vi "Client Output Test.vi"() -> (0 "Error Out":errorcluster, 2 "Pass?":bool)   [LabVIEW 2013, in "OPC UA Client Tests.lvlib"]
doc: "Test functionality of output.vi of the OPC UA Client runtime.lvclass"
uses:
  OPC UA Client Tests.lvlib
  <vilib>/NI/Tag Bus Module Framework/channel/channel classification.ctl
  module/execution/OPC UA Client runtime.lvclass/OPC UA Client runtime.ctl
  module/execution/OPC UA Client runtime.lvclass
  <vilib>/NI/Tag Bus Module Framework/channel/TBM channel.lvclass
panel:
  out "Individual Tests":bool[](array[boolean])
  # "13"
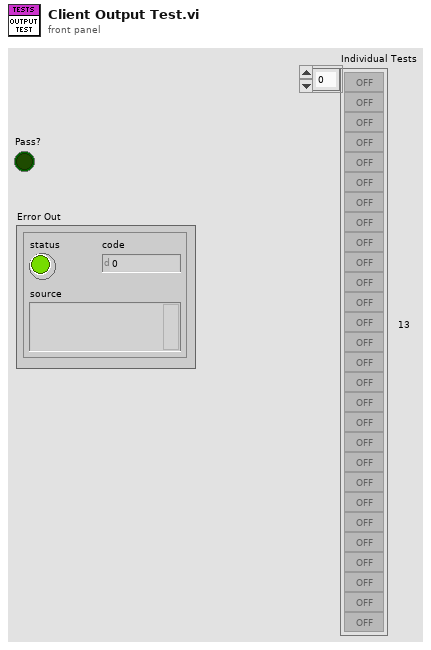
[diagram p1: front panel]
types:
  T1 = typedef "TBM channel.lvclass/channel classification.ctl" = enum16{"input data", "output data", "processing parameter", "processing result"}
  T2 = typedef "TBM channel.lvclass/data tables.ctl" = cluster{"input data":T3, "processing parameter":T3, "processing result":T3, "output data":T3}
  T3 = typedef "tag bus.lvlib/dictionary table pair.ctl" = cluster{"data dictionary":refnum<class "data dictionary.lvclass">, "data table":T4}
  T4 = typedef "tag bus.lvlib/data table.lvlib/data table.ctl" = cluster{"Double":dbl[], "Single":sgl[], "I64":i64[], "I32":i32[], "I16":i16[], "I8":i8[], "U64":u64[], "U32":u32[], "U16":u16[], "U8":u8[], "Boolean":bool[], "String":string[], "Array of Double":cluster{"DBL Array":dbl[]}[], "Array of Single":cluster{"SGL Array":sgl[]}[], "Array of I64":cluster{"I64 Array":i64[]}[], "Array of I32":cluster{"I32 Array":i32[]}[], "Array of I16":cluster{"I16 Array":i16[]}[], "Array of I8":cluster{"I8 Array":i8[]}[], "Array of U64":cluster{"U64 Array":u64[]}[], "Array of U32":cluster{"U32 Array":u32[]}[], "Array of U16":cluster{"U16 Array":u16[]}[], "Array of U8":cluster{"U8 Array":u8[]}[], "Array of Boolean":cluster{"Boolean Array":bool[]}[], "Array of String":cluster{"String Array":string[]}[]}
  T5 = typedef "OPC UA Client configuration.lvclass/Line.ctl" = cluster{"channel":refnum<class "TBM channel.lvclass">, "Node Path":string, "OPC UA Data Type":T6}
  T6 = typedef "OPC UA Client configuration.lvclass/OPC UA Data Type.ctl" = u16
  T7 = typedef "tag bus.lvlib/tag descriptor.lvclass/Data Type.ctl" = enum16{"Double", "Single", "I64", "I32", "I16", "I8", "U64", "U32", "U16", "U8", "Boolean", "String", "Array of Double", "Array of Single", "Array of I64", "Array of I32", "Array of I16", "Array of I8", "Array of U64", "Array of U32", "Array of U16", "Array of U8", "Array of Boolean", "Array of String"}
  T8 = cluster{"DCAF Data Type":T7, "Index":i32, "Node Path":string, "OPC UA Data Type":T6}[]
  T9 = cluster{"Node Path":string, "Flattened Data":string}[]
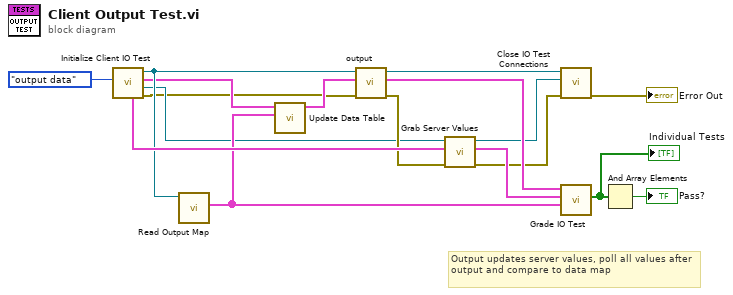
[diagram p0: block diagram]
diagram:
  # "Output updates server values, poll all values after output and compare to data map"
  n1 = call "Initialize Client IO Test.vi"("channel classification"=channel_classification."output data") -> ("error out"=w1:errorcluster, "OPC UA server refnum out"=w3:refnum<k21>, "data allocations"=w10:T2, "OPC UA runtime out"=w12:refnum<class "OPC UA Client runtime.lvclass">, "Lines"=w16:T5[])  [unwired: 6 in]
  n2 = call "Read Output Map.vi"("OPC UA Client runtime in"=w12) -> ("Output Map"=w11:T8)  [unwired: 9 in, 1 out]
  n3 = call "Update Data Table.vi"("Output Map"=w11, "data allocations"=w10) -> ("data table out"=w9:T4)  [unwired: 9 in]
  n4 = call-dynamic "output.vi"("error in"=w1, "data table in"=w9, "OPC UA runtime in"=w12) -> ("error out"=w8:errorcluster, "data table out"=w15:T4, "OPC UA runtime out"=w14:refnum<class "OPC UA Client runtime.lvclass">)  [unwired: 6 in]
  n5 = call "Grab Server Values.vi"("error in (no error)"=w8, "Lines"=w16, "OPC UA server refnum"=w3) -> ("error out"=w7:errorcluster, "Server Data"=w13:T9, "OPC UA server refnum"=w2:refnum<k21>)  [unwired: 4 in]
  n6 = call "Close IO Test Connections.vi"("error in"=w7, "OPC UA server refnum"=w2, "OPC UA runtime in"=w14) -> ("error out"=→"Error Out":errorcluster)  [unwired: 8 in]
  n7 = call "Grade IO Test.vi"("Data Map"=w11, "Server Data"=w13, "data table in"=w15) -> ("Pass?"=w5:bool[])  [unwired: 7 in]
  "Individual Tests" <- w5
  n8 = And Array Elements(Boolean array=w5) -> (logical AND=→"Pass?":bool)
